vi "Add Groups to Tree.vi"(8 "error in":errorcluster, 10 "Tree Items Parent":string, 11 "Report Viewer in":refnum<class "Report Viewer.lvclass">) -> (0 "error out":errorcluster, 2 "Group_Based_Items":string[](array[string]), 3 "Report Viewer out":refnum<class "Report Viewer.lvclass">)   [LabVIEW 2023, in "Report Viewer.lvlib" / "Report Viewer.lvclass"]
uses:
  Library/Report Viewer.lvclass
  Library/Report Viewer.lvclass/Report Viewer.ctl
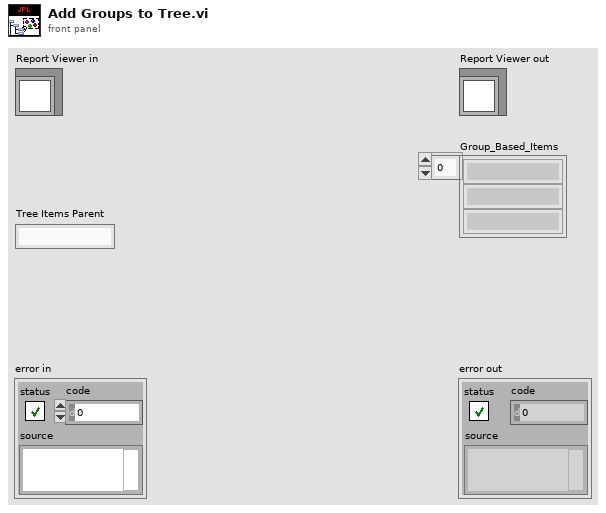
[diagram p1: front panel]
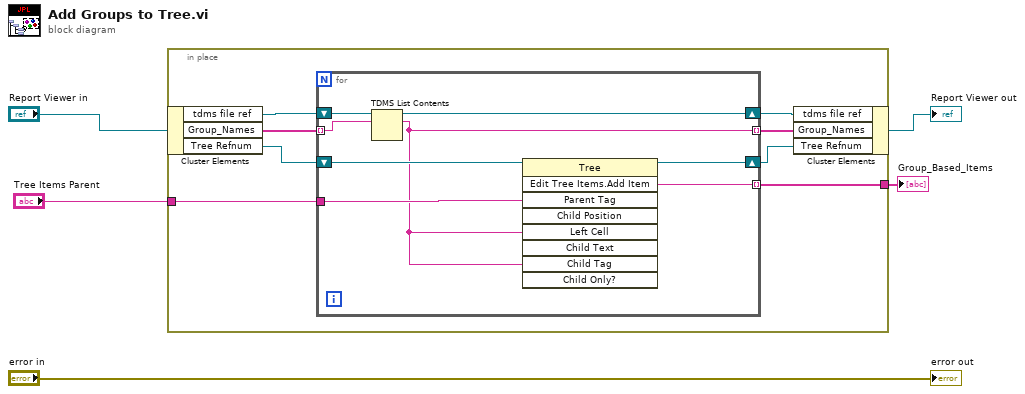
[diagram p0: block diagram]
diagram:
  n1 = in-place {
    in-place-border: "Tree Items Parent" -> [w7]
    in-place-border: [w6] -> w1
    n2 = in-place-cluster #1("Report Viewer in") -> ("tdms file ref"=w13:refnum<k34>, "Group_Names"=w11:string[], "Tree Refnum"=w9:refnum<vi>)
    n3 = for {
      shift-right: [w20] -> w12
      shift-left: w13 -> [w21]
      tunnel: w11 -> [w19] mode=indexing
      tunnel: [w14] -> w10 mode=indexing
      shift-right: [w17] -> w8
      shift-left: w9 -> [w18]
      tunnel: w7 -> [w16]
      tunnel: [w15] -> w6 mode=indexing
      n4 = TDMS List Contents(6:w19, 7:w21) -> (2:w14:string, 3:w20:refnum<k34>)  [unwired: 1 in, 2 out]
      n5 = invoke on="Invoke Node" class="Tree" method="Edit Tree Items.Add Item"(reference=w18, "Parent Tag"=w16, "Left Cell"=w14, "Child Tag"=w14) -> (reference out=w17:refnum<vi>, "Edit Tree Items:Add Item"=w15:string)  [unwired: 5 in, 7 out]
    }
    n6 = in-place-cluster #1("tdms file ref"=w12, "Group_Names"=w10, "Tree Refnum"=w8) -> (→"Report Viewer out":refnum<class "Report Viewer.lvclass">)
  }
  "Group_Based_Items" <- w1
  "error out" <- "error in"
